vi "System Time Resolution Test.vi"() -> ()   [LabVIEW 2021]
panel:
  out "Array":u32[](array[numeric])
  # "Use this to see if the resolution of the system timer, and make sure it is 1 ms\nand not 16 ms.\n\nIf I put in a time interval of 1 ms, my system time stamps increment by 2 ms.\n\nIf I put in a time interval of 0, I had to tell it to iterate 1000 times, and around\niteration 900 finally saw the clock increment by 1 ms."
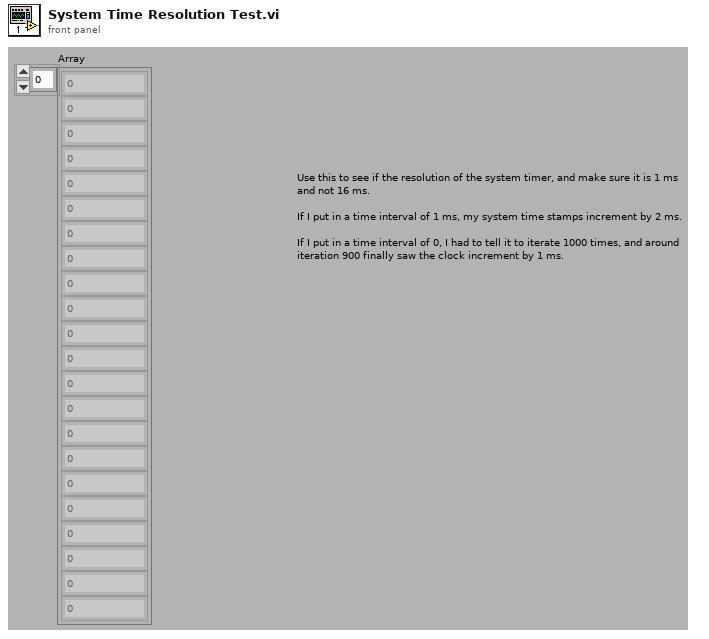
[diagram p1: front panel]
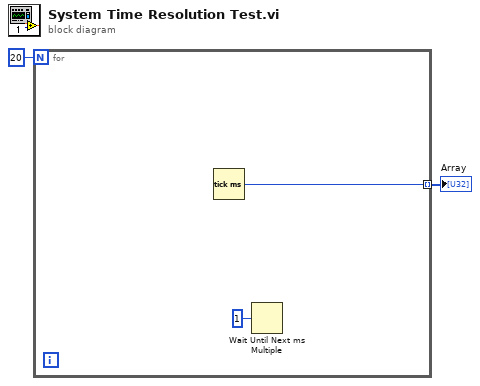
[diagram p0: block diagram]
diagram:
  n1 = for {
    N: 20 -> [_]
    tunnel: [w4] -> w1 mode=indexing
    n2 = Tick Count (ms)() -> (millisecond timer value=w4:u32)
    n3 = Wait Until Next ms Multiple(millisecond multiple=u32 1) -> ()  [unwired: 1 out]
  }
  "Array" <- w1
